vi "Add Multiple.vi"(6 "Input Settings":T1, 7 "Settings":T3, 8 "error in (no error)":errorcluster, 9 "Fixtures":T2[](array[typedef]), 10 "Routine":T4[](array[typedef]), 11 "Assembly in":refnum<class "Assembly Run.lvclass">) -> (0 "error out":errorcluster, 3 "Assembly out":refnum<class "Assembly Run.lvclass">)   [LabVIEW 2021, in "Assembly Run.lvclass"]
uses:
  Assembly Run.lvclass
  Routine/Routine Enum.ctl
  Routine/Settings.ctl
  Workspace/Fixture Enum.ctl
  Routine/Routine.lvclass
  Workspace/Fixture.lvclass
panel:
  in  "Assembly Type":string
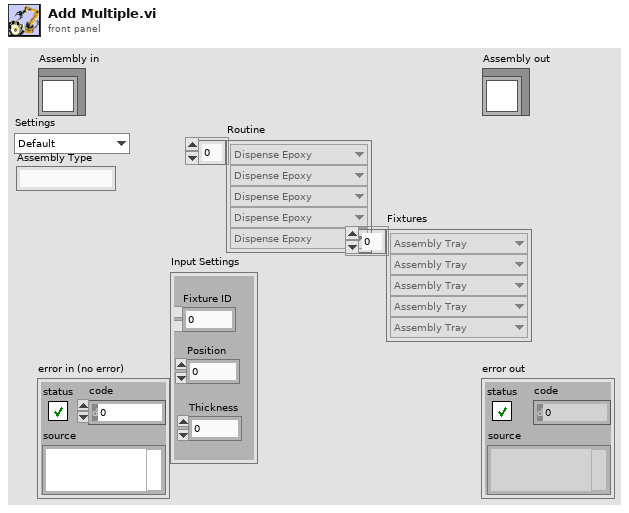
[diagram p1: front panel]
types:
  T1 = cluster{"Fixture ID":dbl, "Position":dbl, "Thickness":dbl}
  T2 = typedef "Fixture.lvclass/Fixture Enum.ctl" = enum16{"Assembly Tray", "Syringe Space", "Component", "Pick Up Tool", "Current Position"}
  T3 = typedef "Routine.lvclass/Settings.ctl" = enum16{"Default", "Custom"}
  T4 = typedef "Routine.lvclass/Routine Enum.ctl" = enum16{"Primary Pick Up", "Secondary Pick Up", "Put Down All", "Secure Syringe", "Release Syringe", "Dispense Epoxy", "Pick Up All", "Put Down Secondary", "Full Assembly"}
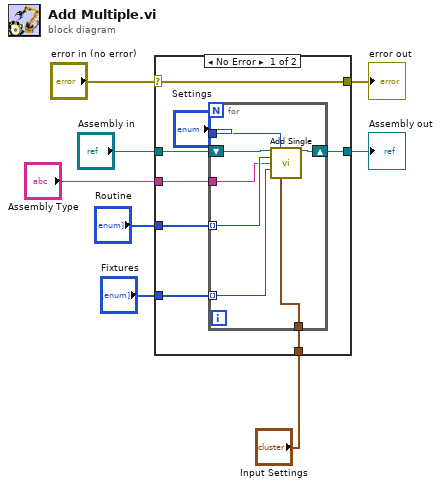
[diagram p0: block diagram]
diagram:
  n1 = case shown="No Error" "error in (no error)" {
    selector: "error in (no error)" -> [w16 w25]
    tunnel: [w16 w25] -> w7
    tunnel: [w14 w24] -> w5
    tunnel: "Assembly in" -> [w15 w24]
    tunnel: "Routine" -> [w13 _]
    tunnel: "Fixtures" -> [w11 _]
    tunnel: "Input Settings" -> [w10 _]
    tunnel: "Assembly Type" -> [w9 _]
    frame No Error {
      n2 = for {
        shift-right: [w20] -> w14
        shift-left: w15 -> [w22]
        tunnel: w13 -> [w19] mode=indexing
        tunnel: "Settings" -> [w21]
        tunnel: w11 -> [w23] mode=indexing
        tunnel: w10 -> [w18]
        tunnel: w9 -> [w17]
        n3 = call-dynamic "Add Single.vi"("UI in"=w22, "Settings"=w21, "Routine"=w19, "Assembly Type"=w17, "Fixture"=w23, "Input Settings"=w18) -> ("UI out"=w20:refnum<class "Assembly Run.lvclass">)  [unwired: 8 in, 1 out]
      }
    }
    frame Error {
    }
  }
  "error out" <- w7
  "Assembly out" <- w5
